vi "syringe_pump_tester.vi"() -> ()   [LabVIEW 2018]
panel:
  in  "Max Pull":bool
  in  "Max Push":bool
  in  "Stop Hold":bool
  out "System Status":T1={"pumpState"=2, "pumpError"=0, "suppliedVolume_ml"=nan, "flowRate_mlmin"=0.0}
  in  "Flow Config":T2={"direction"=1, "desVolume_ml"=5.0, "desFlowrate_mlpmin"=5.0, "syringeDiameter_mm"=20.0}
  in  "Hardware Config":T3={"pwmFrequency"=0, "pwmSlope"=0, "pwmJitter"=0, "stepMode"=32, "maxDriverCurrent_mA"=850, "stepsPerRev"=400, "leadScrewPitch_mm"=1.5, "maxPullPushAcc_RevPerSecSec"=4.0, "maxPullPushVel_RevPerSec"=4.0, "pumpAcc_RevPerSecSec"=0.1, "pumpDec_RevPerSecSec"=0.1}
  in  "Apply Hardware Config":bool
  in  "Apply Flow Config":bool
  in  "Stop Pump":bool
  in  "Start Pump":bool
  out "Error Code":T4(ring)
  out "Return FID":u8=1
  out "FID":u8=1
  in  "IP Address":string="192.168.5.104"
  out "error out":errorcluster={"status"=TRUE, "code"=56, "source"="TCP Open Connection in syringe_pump_tester.vi"}
  in  "Get System Status":bool
  in  "Stop":bool
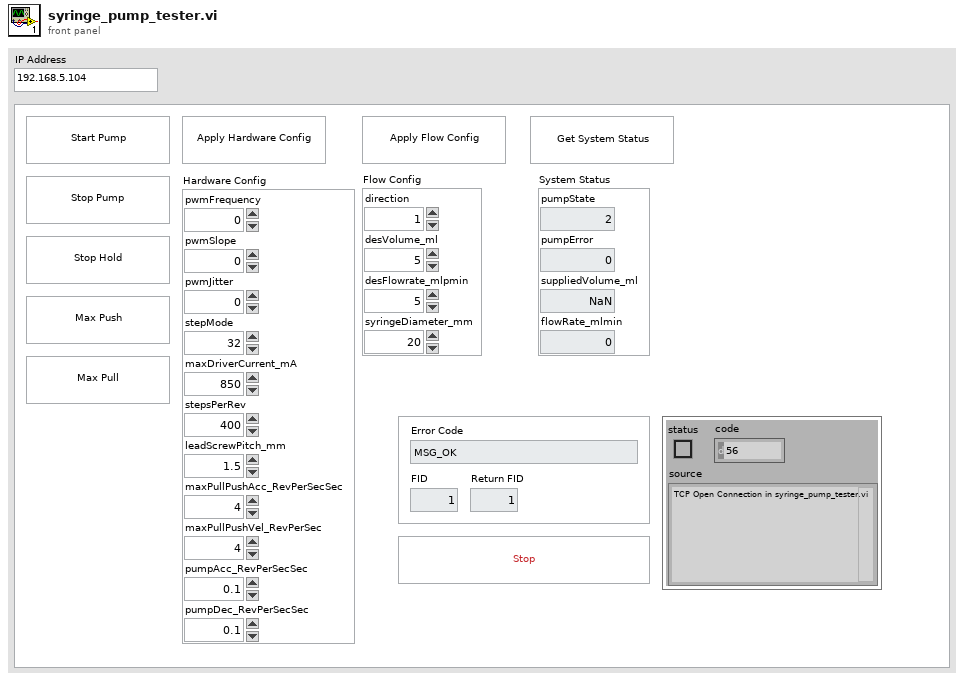
[diagram p1: front panel]
types:
  T1 = cluster{"pumpState":i32, "pumpError":i32, "suppliedVolume_ml":sgl, "flowRate_mlmin":sgl}
  T2 = cluster{"direction":u8, "desVolume_ml":sgl, "desFlowrate_mlpmin":sgl, "syringeDiameter_mm":sgl}
  T3 = cluster{"pwmFrequency":u8, "pwmSlope":u8, "pwmJitter":u8, "stepMode":u8, "maxDriverCurrent_mA":u16, "stepsPerRev":i32, "leadScrewPitch_mm":sgl, "maxPullPushAcc_RevPerSecSec":sgl, "maxPullPushVel_RevPerSec":sgl, "pumpAcc_RevPerSecSec":sgl, "pumpDec_RevPerSecSec":sgl}
  T4 = enum16{"MSG_OK", "MSG_ERROR_INVALID_PARAMETER", "MSG_ERROR_NOT_SUPPORTED", "MSG_ERROR_PUMP_RUNNING", "MSG_ERROR_CHECK_POWER", "MSG_ERROR_FLOW_NOT_CONFIGURED", "MSG_ERROR_STEPDRV_NOT_CONFIGURED", "MSG_ERROR_LIMIT_SW_ACTIVE", "MSG_ERROR_STEPDRV_ERROR", "MSG_ERROR_NO_I2C_COM", "MSG_ERROR_SWITCHING_OVER_MAX"}
  T5 = enum16{"big-endian, network order", "native, host order", "little-endian"}
  T6 = cluster{"connection ID":refnum<k5>, "header length":i32}
  T7 = cluster{"header":cluster{"length":u8, "fid":u8, "error":u8}}
  T8 = cluster{"header":cluster{"length":u8, "fid":u8, "error":u8}, "Hardware Config":cluster{"pwmFrequency":u8, "pwmSlope":u8, "pwmJitter":u8, "stepMode":u8, "maxDriverCurrent_mA":u16, "stepsPerRev":i32, "leadScrewPitch_mm":sgl, "maxPullPushAcc_RevPerSecSec":sgl, "maxPullPushVel_RevPerSec":sgl, "pumpAcc_RevPerSecSec":sgl, "pumpDec_RevPerSecSec":sgl}}
  T9 = cluster{"header":cluster{"length":u8, "fid":u8, "error":u8}, "Flow Config":cluster{"direction":u8, "desVolume_ml":sgl, "desFlowrate_mlpmin":sgl, "syringeDiameter_mm":sgl}}
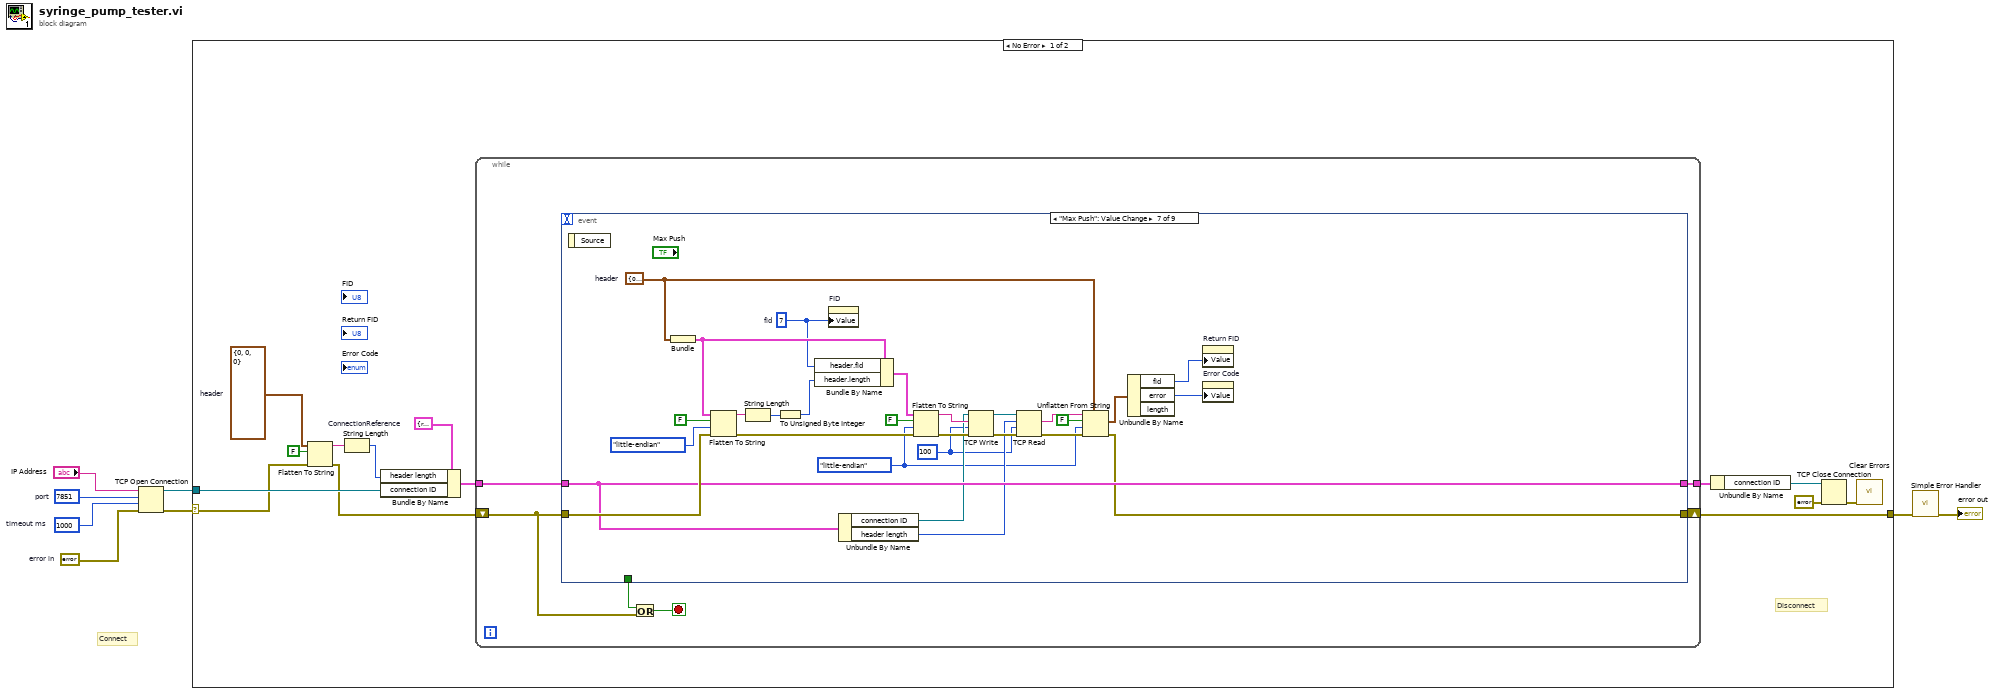
[diagram p0: block diagram]
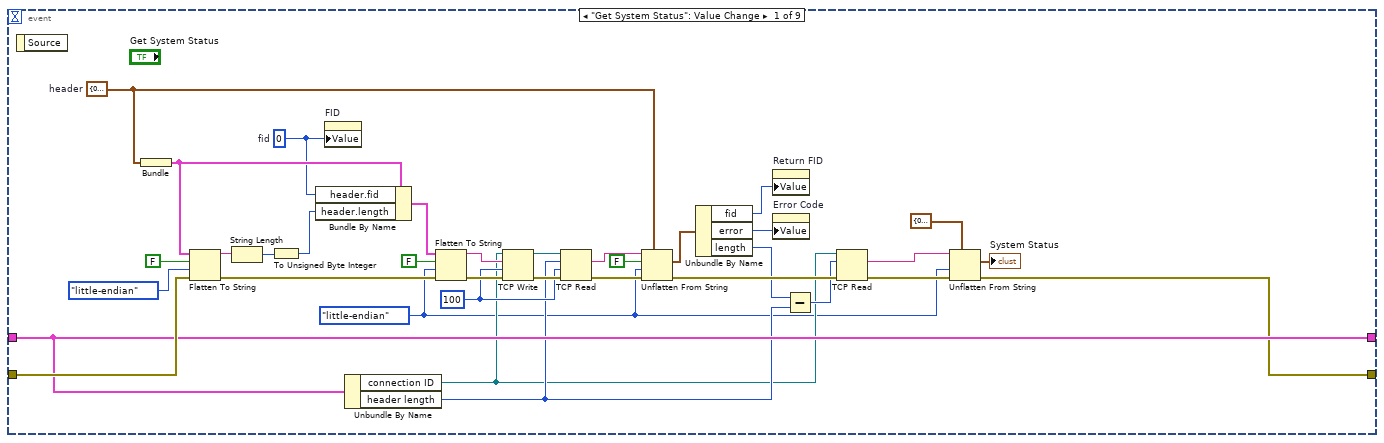
[diagram p2: hidden frame]
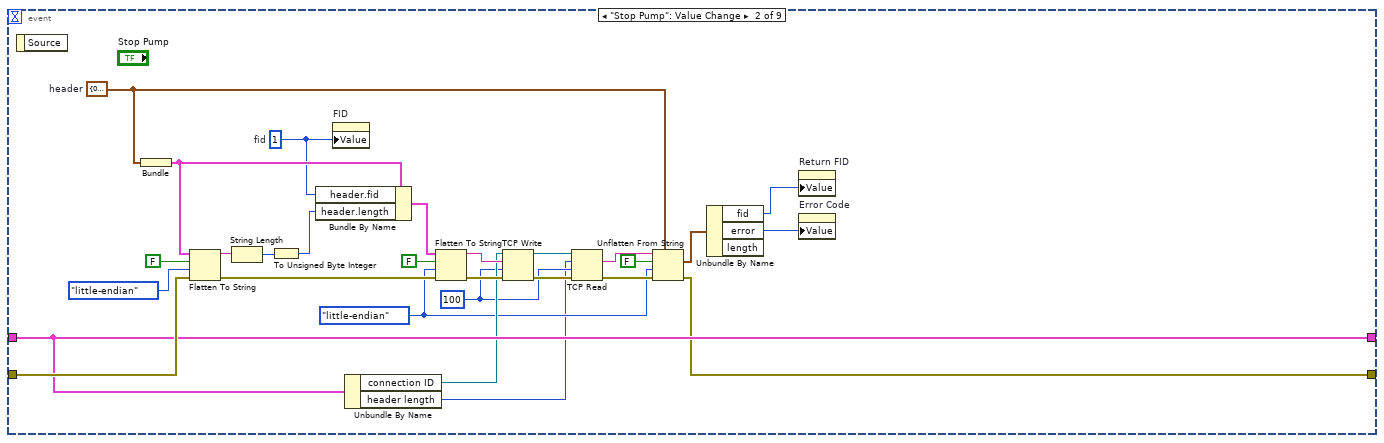
[diagram p3: hidden frame]
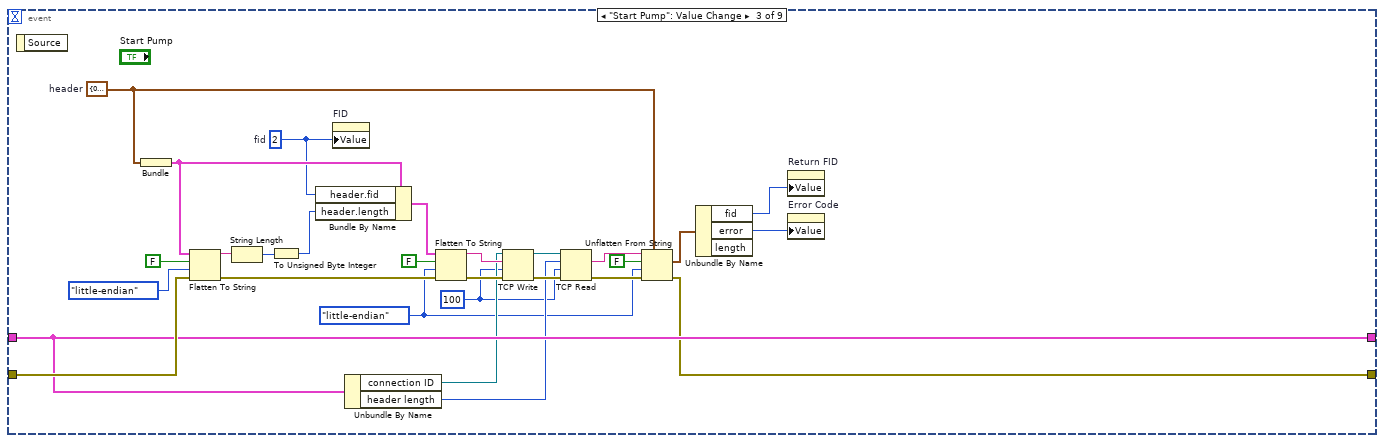
[diagram p4: hidden frame]
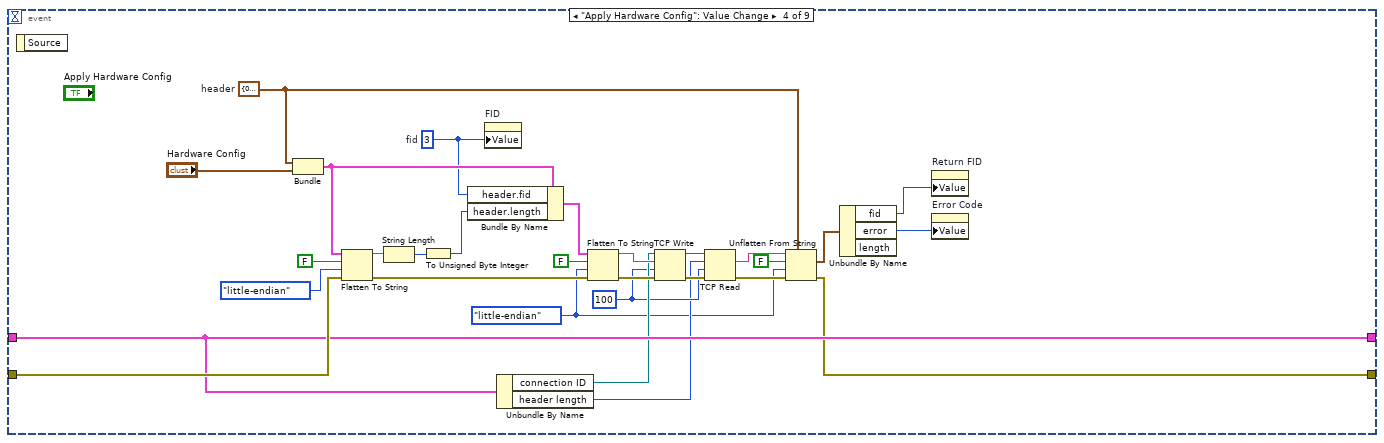
[diagram p5: hidden frame]
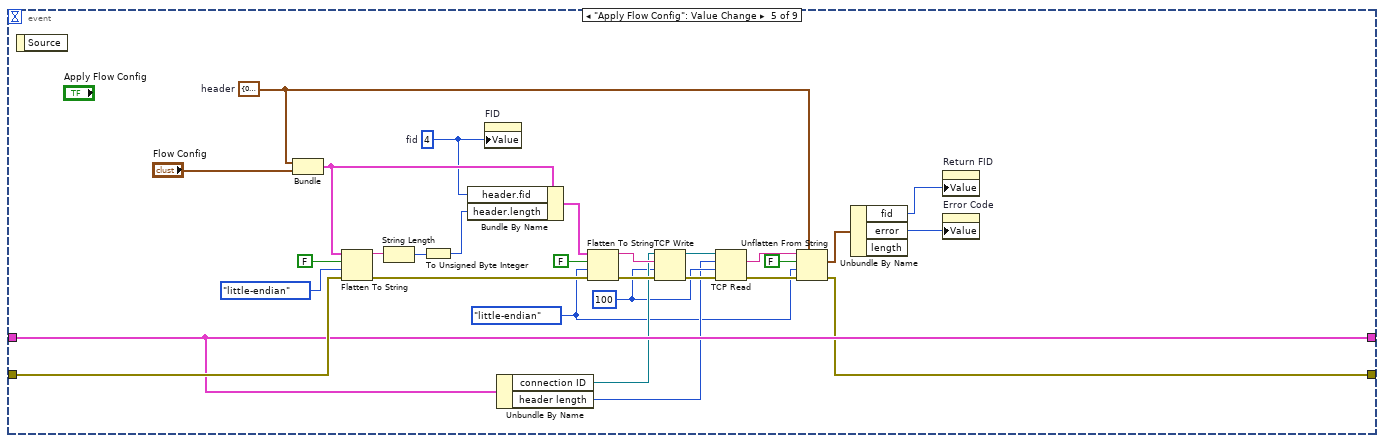
[diagram p6: hidden frame]
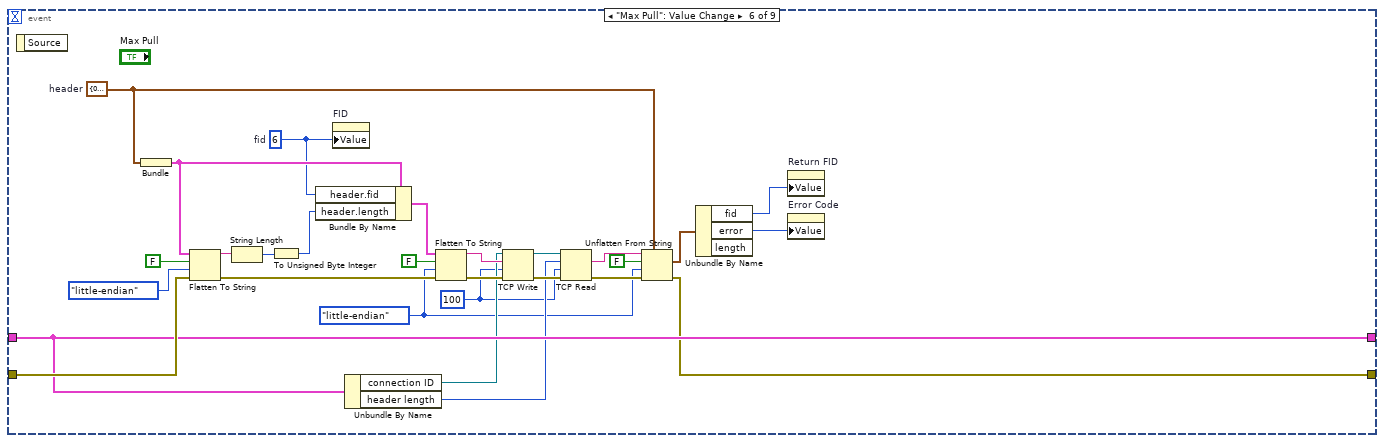
[diagram p7: hidden frame]
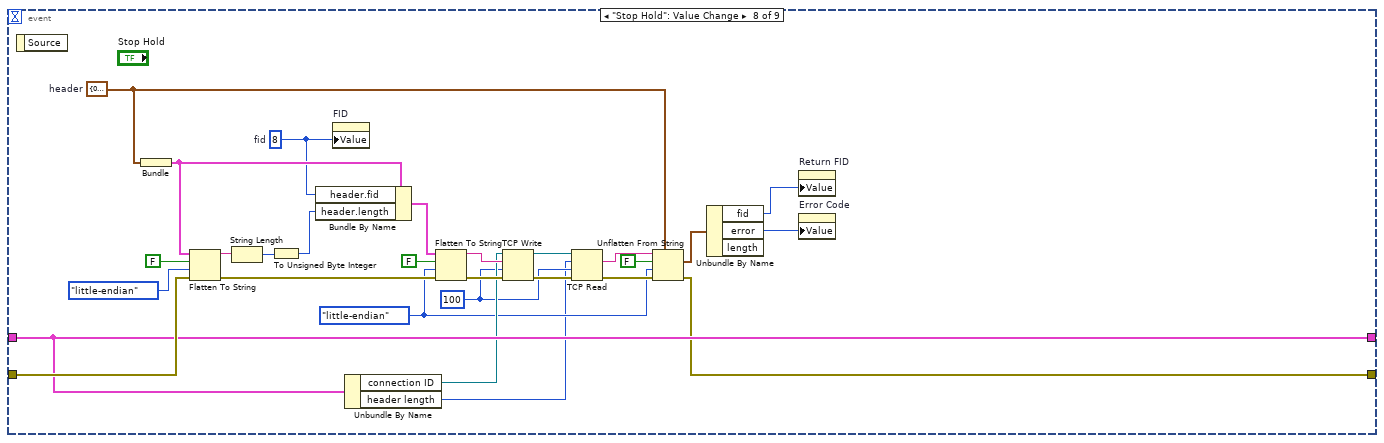
[diagram p8: hidden frame]
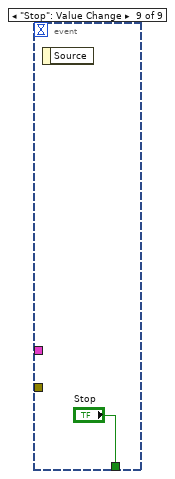
[diagram p9: hidden frame]
diagram:
  w6 = errorcluster {"status"=FALSE, "code"=0, "source"=""}  # error in
  w7 = 1000  # timeout ms
  w8 = u16 7851  # port
  # "Connect"
  n1 = TCP Open Connection(address="IP Address", remote port or service name=w8, timeout ms (60000)=w7, error in (no error)=w6) -> (connection ID=w5:refnum<k5>, error out=w1:errorcluster)  [unwired: 1 in]
  n2 = case shown="No Error" w1 {
    selector: w1 -> [w9 w263]
    tunnel: w5 -> [w18 _]
    tunnel: [w10 w263] -> w2
    frame No Error {
      w17 = cluster{"length":u8, "fid":u8, "error":u8} {"length"=0, "fid"=0, "error"=0}  # header
      w19 = T6 {"connection ID"=refnum, "header length"=0}  # ConnectionReference
      # "Disconnect"
      n3 = Flatten To String(anything=w17, prepend array or string size? (T)=FALSE, error in (no error)=w9) -> (data string=w15:string, error out=w11:errorcluster)  [unwired: 1 in, 1 out]
      n4 = String Length(string=w15) -> (length=w14:i32)
      n5 = Bundle By Name(cluster=w19, "header length"=w14, "connection ID"=w18) -> (w13:T6)
      n6 = while {
        tunnel: w13 -> [w28]
        tunnel: [w27] -> w12
        shift-right: [w26] -> w10
        shift-left: w11 -> [w24]
        stop <- w25 stop-if-true
        n7 = event shown="[6] \"Max Push\": Value Change" {
          selector: _ -> [_ _ _ _ _ _ _ _ _]
          dyn-events: _ -> [_ _ _ _ _ _ _ _ _]
          timeout: _ -> [_ _ _ _ _ _ _ _ _]
          tunnel: w28 -> [w52 w80 w108 w137 w166 w194 w222 w250 _]
          tunnel: [w52 w80 w108 w137 w166 w194 w222 w250 _] -> w27
          tunnel: w24 -> [w53 w81 w109 w138 w167 w195 w223 w251 _]
          tunnel: [w35 w71 w92 w123 w150 w178 w206 w241 _] -> w26
          tunnel: [_ _ _ _ _ _ _ _ "Stop"] -> w23
          event "Get System Status": Value Change {
            w44 = cluster{"length":u8, "fid":u8, "error":u8} {"length"=0, "fid"=0, "error"=0}  # header
            w46 = 100 ("timeout ms (25000)")
            w32 = u8 0  # fid
            w34 = T5."little-endian" ("byte order (0:big-endian, network order)")
            n8 = event-data() -> ()  [unwired: 1 in, 1 out]
            n9 = Bundle("header"=w44) -> (w59:T7)  [unwired: 1 in]
            n10 = Flatten To String(anything=w59, prepend array or string size? (T)=FALSE, byte order (0:big-endian, network order)=T5."little-endian", error in (no error)=w53) -> (data string=w57:string, error out=w58:errorcluster)  [unwired: 1 out]
            n11 = String Length(string=w57) -> (length=w56:i32)
            n12 = To Unsigned Byte Integer(number=w56) -> (unsigned 8bit integer=w55:u8)
            n13 = Bundle By Name(cluster=w59, "header.fid"=w32, "header.length"=w55) -> (w60:T7)
            n14 = property on="FID" class="DigNum (strict)"("Value"=w32) -> ()  [unwired: 2 in, 2 out]
            n15 = Unbundle By Name(w52) -> ("connection ID"=w38:refnum<k5>, "header length"=w40:i32)
            n16 = Flatten To String(anything=w60, prepend array or string size? (T)=FALSE, byte order (0:big-endian, network order)=w34, error in (no error)=w58) -> (data string=w62:string, error out=w63:errorcluster)  [unwired: 1 out]
            n17 = TCP Write(connection ID=w38, data in=w62, error in (no error)=w63, 9:w46) -> (connection ID out=w47:refnum<k5>, error out=w48:errorcluster)  [unwired: 1 out]
            n18 = TCP Read(connection ID=w47, bytes to read=w40, error in (no error)=w48, 9:w46) -> (data out=w49:string, error out=w50:errorcluster)  [unwired: 1 in, 1 out]
            n19 = Unflatten From String(type=w44, binary string=w49, data includes array or string size? (T)=FALSE, byte order (0:big-endian, network order)=w34, error in (no error)=w50) -> (value=w45:cluster{"length":u8, "fid":u8, "error":u8}, error out=w42:errorcluster)  [unwired: 1 out]
            n20 = Unbundle By Name(w45) -> ("fid"=w33:u8, "error"=w31:u8, "length"=w41:u8)
            n21 = property on="Return FID" class="DigNum (strict)"("Value"=w33) -> ()  [unwired: 2 in, 2 out]
            n22 = property on="Error Code" class="Enum (strict)"("Value"=w31) -> ()  [unwired: 2 in, 2 out]
            n23 = Subtract(x=w41, y=w40) -> (x-y=w39:i32)
            n24 = TCP Read(connection ID=w38, bytes to read=w39, error in (no error)=w42) -> (data out=w37:string, error out=w36:errorcluster)  [unwired: 2 in, 1 out]
            n25 = Unflatten From String(type=T1 {"pumpState"=0, "pumpError"=0, "suppliedVolume_ml"=0.0, "flowRate_mlmin"=0.0} ("system status"), binary string=w37, byte order (0:big-endian, network order)=w34, error in (no error)=w36) -> (value=→"System Status":T1, error out=w35:errorcluster)  [unwired: 1 in, 1 out]
          }
          event "Stop Pump": Value Change {
            w70 = cluster{"length":u8, "fid":u8, "error":u8} {"length"=0, "fid"=0, "error"=0}  # header
            w68 = 100 ("timeout ms (25000)")
            w77 = u8 1  # fid
            w69 = T5."little-endian" ("byte order (0:big-endian, network order)")
            n26 = event-data() -> ()  [unwired: 1 in, 1 out]
            n27 = Bundle("header"=w70) -> (w87:T7)  [unwired: 1 in]
            n28 = Flatten To String(anything=w87, prepend array or string size? (T)=FALSE, byte order (0:big-endian, network order)=T5."little-endian", error in (no error)=w81) -> (data string=w85:string, error out=w86:errorcluster)  [unwired: 1 out]
            n29 = String Length(string=w85) -> (length=w84:i32)
            n30 = To Unsigned Byte Integer(number=w84) -> (unsigned 8bit integer=w83:u8)
            n31 = Bundle By Name(cluster=w87, "header.fid"=w77, "header.length"=w83) -> (w88:T7)
            n32 = property on="FID" class="DigNum (strict)"("Value"=w77) -> ()  [unwired: 2 in, 2 out]
            n33 = Unbundle By Name(w80) -> ("connection ID"=w78:refnum<k5>, "header length"=w67:i32)
            n34 = Flatten To String(anything=w88, prepend array or string size? (T)=FALSE, byte order (0:big-endian, network order)=w69, error in (no error)=w86) -> (data string=w90:string, error out=w91:errorcluster)  [unwired: 1 out]
            n35 = TCP Write(connection ID=w78, data in=w90, error in (no error)=w91, 9:w68) -> (connection ID out=w66:refnum<k5>, error out=w73:errorcluster)  [unwired: 1 out]
            n36 = TCP Read(connection ID=w66, bytes to read=w67, error in (no error)=w73, 9:w68) -> (data out=w76:string, error out=w72:errorcluster)  [unwired: 1 in, 1 out]
            n37 = Unflatten From String(type=w70, binary string=w76, data includes array or string size? (T)=FALSE, byte order (0:big-endian, network order)=w69, error in (no error)=w72) -> (value=w75:cluster{"length":u8, "fid":u8, "error":u8}, error out=w71:errorcluster)  [unwired: 1 out]
            n38 = Unbundle By Name(w75) -> ("fid"=w65:u8, "error"=w64:u8)  [unwired: 1 out]
            n39 = property on="Return FID" class="DigNum (strict)"("Value"=w65) -> ()  [unwired: 2 in, 2 out]
            n40 = property on="Error Code" class="Enum (strict)"("Value"=w64) -> ()  [unwired: 2 in, 2 out]
          }
          event "Start Pump": Value Change {
            w101 = cluster{"length":u8, "fid":u8, "error":u8} {"length"=0, "fid"=0, "error"=0}  # header
            w93 = 100 ("timeout ms (25000)")
            w97 = u8 2  # fid
            w94 = T5."little-endian" ("byte order (0:big-endian, network order)")
            n41 = event-data() -> ()  [unwired: 1 in, 1 out]
            n42 = Bundle("header"=w101) -> (w115:T7)  [unwired: 1 in]
            n43 = Flatten To String(anything=w115, prepend array or string size? (T)=FALSE, byte order (0:big-endian, network order)=T5."little-endian", error in (no error)=w109) -> (data string=w113:string, error out=w114:errorcluster)  [unwired: 1 out]
            n44 = String Length(string=w113) -> (length=w112:i32)
            n45 = To Unsigned Byte Integer(number=w112) -> (unsigned 8bit integer=w111:u8)
            n46 = Bundle By Name(cluster=w115, "header.fid"=w97, "header.length"=w111) -> (w116:T7)
            n47 = property on="FID" class="DigNum (strict)"("Value"=w97) -> ()  [unwired: 2 in, 2 out]
            n48 = Unbundle By Name(w108) -> ("connection ID"=w98:refnum<k5>, "header length"=w99:i32)
            n49 = Flatten To String(anything=w116, prepend array or string size? (T)=FALSE, byte order (0:big-endian, network order)=w94, error in (no error)=w114) -> (data string=w118:string, error out=w119:errorcluster)  [unwired: 1 out]
            n50 = TCP Write(connection ID=w98, data in=w118, error in (no error)=w119, 9:w93) -> (connection ID out=w103:refnum<k5>, error out=w104:errorcluster)  [unwired: 1 out]
            n51 = TCP Read(connection ID=w103, bytes to read=w99, error in (no error)=w104, 9:w93) -> (data out=w105:string, error out=w106:errorcluster)  [unwired: 1 in, 1 out]
            n52 = Unflatten From String(type=w101, binary string=w105, data includes array or string size? (T)=FALSE, byte order (0:big-endian, network order)=w94, error in (no error)=w106) -> (value=w102:cluster{"length":u8, "fid":u8, "error":u8}, error out=w92:errorcluster)  [unwired: 1 out]
            n53 = Unbundle By Name(w102) -> ("fid"=w96:u8, "error"=w95:u8)  [unwired: 1 out]
            n54 = property on="Return FID" class="DigNum (strict)"("Value"=w96) -> ()  [unwired: 2 in, 2 out]
            n55 = property on="Error Code" class="Enum (strict)"("Value"=w95) -> ()  [unwired: 2 in, 2 out]
          }
          event "Apply Hardware Config": Value Change {
            w126 = cluster{"length":u8, "fid":u8, "error":u8} {"length"=0, "fid"=0, "error"=0}  # header
            w127 = 100 ("timeout ms (25000)")
            w134 = u8 3  # fid
            w120 = T5."little-endian" ("byte order (0:big-endian, network order)")
            n56 = event-data() -> ()  [unwired: 1 in, 1 out]
            n57 = Bundle("header"=w126, "Hardware Config"="Hardware Config") -> (w144:T8)  [unwired: 1 in]
            n58 = Flatten To String(anything=w144, prepend array or string size? (T)=FALSE, byte order (0:big-endian, network order)=T5."little-endian", error in (no error)=w138) -> (data string=w142:string, error out=w143:errorcluster)  [unwired: 1 out]
            n59 = String Length(string=w142) -> (length=w141:i32)
            n60 = To Unsigned Byte Integer(number=w141) -> (unsigned 8bit integer=w140:u8)
            n61 = Bundle By Name(cluster=w144, "header.fid"=w134, "header.length"=w140) -> (w145:T8)
            n62 = property on="FID" class="DigNum (strict)"("Value"=w134) -> ()  [unwired: 2 in, 2 out]
            n63 = Unbundle By Name(w137) -> ("connection ID"=w135:refnum<k5>, "header length"=w124:i32)
            n64 = Flatten To String(anything=w145, prepend array or string size? (T)=FALSE, byte order (0:big-endian, network order)=w120, error in (no error)=w143) -> (data string=w147:string, error out=w148:errorcluster)  [unwired: 1 out]
            n65 = TCP Write(connection ID=w135, data in=w147, error in (no error)=w148, 9:w127) -> (connection ID out=w125:refnum<k5>, error out=w128:errorcluster)  [unwired: 1 out]
            n66 = TCP Read(connection ID=w125, bytes to read=w124, error in (no error)=w128, 9:w127) -> (data out=w131:string, error out=w132:errorcluster)  [unwired: 1 in, 1 out]
            n67 = Unflatten From String(type=w126, binary string=w131, data includes array or string size? (T)=FALSE, byte order (0:big-endian, network order)=w120, error in (no error)=w132) -> (value=w130:cluster{"length":u8, "fid":u8, "error":u8}, error out=w123:errorcluster)  [unwired: 1 out]
            n68 = Unbundle By Name(w130) -> ("fid"=w122:u8, "error"=w121:u8)  [unwired: 1 out]
            n69 = property on="Return FID" class="DigNum (strict)"("Value"=w122) -> ()  [unwired: 2 in, 2 out]
            n70 = property on="Error Code" class="Enum (strict)"("Value"=w121) -> ()  [unwired: 2 in, 2 out]
          }
          event "Apply Flow Config": Value Change {
            w153 = cluster{"length":u8, "fid":u8, "error":u8} {"length"=0, "fid"=0, "error"=0}  # header
            w156 = 100 ("timeout ms (25000)")
            w163 = u8 4  # fid
            w149 = T5."little-endian" ("byte order (0:big-endian, network order)")
            n71 = event-data() -> ()  [unwired: 1 in, 1 out]
            n72 = Bundle("header"=w153, "Flow Config"="Flow Config") -> (w173:T9)  [unwired: 1 in]
            n73 = Flatten To String(anything=w173, prepend array or string size? (T)=FALSE, byte order (0:big-endian, network order)=T5."little-endian", error in (no error)=w167) -> (data string=w171:string, error out=w172:errorcluster)  [unwired: 1 out]
            n74 = String Length(string=w171) -> (length=w170:i32)
            n75 = To Unsigned Byte Integer(number=w170) -> (unsigned 8bit integer=w169:u8)
            n76 = Bundle By Name(cluster=w173, "header.fid"=w163, "header.length"=w169) -> (w174:T9)
            n77 = property on="FID" class="DigNum (strict)"("Value"=w163) -> ()  [unwired: 2 in, 2 out]
            n78 = Unbundle By Name(w166) -> ("connection ID"=w164:refnum<k5>, "header length"=w155:i32)
            n79 = Flatten To String(anything=w174, prepend array or string size? (T)=FALSE, byte order (0:big-endian, network order)=w149, error in (no error)=w172) -> (data string=w176:string, error out=w177:errorcluster)  [unwired: 1 out]
            n80 = TCP Write(connection ID=w164, data in=w176, error in (no error)=w177, 9:w156) -> (connection ID out=w154:refnum<k5>, error out=w157:errorcluster)  [unwired: 1 out]
            n81 = TCP Read(connection ID=w154, bytes to read=w155, error in (no error)=w157, 9:w156) -> (data out=w160:string, error out=w161:errorcluster)  [unwired: 1 in, 1 out]
            n82 = Unflatten From String(type=w153, binary string=w160, data includes array or string size? (T)=FALSE, byte order (0:big-endian, network order)=w149, error in (no error)=w161) -> (value=w159:cluster{"length":u8, "fid":u8, "error":u8}, error out=w150:errorcluster)  [unwired: 1 out]
            n83 = Unbundle By Name(w159) -> ("fid"=w152:u8, "error"=w151:u8)  [unwired: 1 out]
            n84 = property on="Return FID" class="DigNum (strict)"("Value"=w152) -> ()  [unwired: 2 in, 2 out]
            n85 = property on="Error Code" class="Enum (strict)"("Value"=w151) -> ()  [unwired: 2 in, 2 out]
          }
          event "Max Pull": Value Change {
            w187 = cluster{"length":u8, "fid":u8, "error":u8} {"length"=0, "fid"=0, "error"=0}  # header
            w179 = 100 ("timeout ms (25000)")
            w183 = u8 6  # fid
            w180 = T5."little-endian" ("byte order (0:big-endian, network order)")
            n86 = event-data() -> ()  [unwired: 1 in, 1 out]
            n87 = Bundle("header"=w187) -> (w201:T7)  [unwired: 1 in]
            n88 = Flatten To String(anything=w201, prepend array or string size? (T)=FALSE, byte order (0:big-endian, network order)=T5."little-endian", error in (no error)=w195) -> (data string=w199:string, error out=w200:errorcluster)  [unwired: 1 out]
            n89 = String Length(string=w199) -> (length=w198:i32)
            n90 = To Unsigned Byte Integer(number=w198) -> (unsigned 8bit integer=w197:u8)
            n91 = Bundle By Name(cluster=w201, "header.fid"=w183, "header.length"=w197) -> (w202:T7)
            n92 = property on="FID" class="DigNum (strict)"("Value"=w183) -> ()  [unwired: 2 in, 2 out]
            n93 = Unbundle By Name(w194) -> ("connection ID"=w184:refnum<k5>, "header length"=w185:i32)
            n94 = Flatten To String(anything=w202, prepend array or string size? (T)=FALSE, byte order (0:big-endian, network order)=w180, error in (no error)=w200) -> (data string=w204:string, error out=w205:errorcluster)  [unwired: 1 out]
            n95 = TCP Write(connection ID=w184, data in=w204, error in (no error)=w205, 9:w179) -> (connection ID out=w189:refnum<k5>, error out=w190:errorcluster)  [unwired: 1 out]
            n96 = TCP Read(connection ID=w189, bytes to read=w185, error in (no error)=w190, 9:w179) -> (data out=w191:string, error out=w192:errorcluster)  [unwired: 1 in, 1 out]
            n97 = Unflatten From String(type=w187, binary string=w191, data includes array or string size? (T)=FALSE, byte order (0:big-endian, network order)=w180, error in (no error)=w192) -> (value=w188:cluster{"length":u8, "fid":u8, "error":u8}, error out=w178:errorcluster)  [unwired: 1 out]
            n98 = Unbundle By Name(w188) -> ("fid"=w182:u8, "error"=w181:u8)  [unwired: 1 out]
            n99 = property on="Return FID" class="DigNum (strict)"("Value"=w182) -> ()  [unwired: 2 in, 2 out]
            n100 = property on="Error Code" class="Enum (strict)"("Value"=w181) -> ()  [unwired: 2 in, 2 out]
          }
          event "Max Push": Value Change {
            w215 = cluster{"length":u8, "fid":u8, "error":u8} {"length"=0, "fid"=0, "error"=0}  # header
            w207 = 100 ("timeout ms (25000)")
            w211 = u8 7  # fid
            w208 = T5."little-endian" ("byte order (0:big-endian, network order)")
            n101 = event-data() -> ()  [unwired: 1 in, 1 out]
            n102 = Bundle("header"=w215) -> (w229:T7)  [unwired: 1 in]
            n103 = Flatten To String(anything=w229, prepend array or string size? (T)=FALSE, byte order (0:big-endian, network order)=T5."little-endian", error in (no error)=w223) -> (data string=w227:string, error out=w228:errorcluster)  [unwired: 1 out]
            n104 = String Length(string=w227) -> (length=w226:i32)
            n105 = To Unsigned Byte Integer(number=w226) -> (unsigned 8bit integer=w225:u8)
            n106 = Bundle By Name(cluster=w229, "header.fid"=w211, "header.length"=w225) -> (w230:T7)
            n107 = property on="FID" class="DigNum (strict)"("Value"=w211) -> ()  [unwired: 2 in, 2 out]
            n108 = Unbundle By Name(w222) -> ("connection ID"=w212:refnum<k5>, "header length"=w213:i32)
            n109 = Flatten To String(anything=w230, prepend array or string size? (T)=FALSE, byte order (0:big-endian, network order)=w208, error in (no error)=w228) -> (data string=w232:string, error out=w233:errorcluster)  [unwired: 1 out]
            n110 = TCP Write(connection ID=w212, data in=w232, error in (no error)=w233, 9:w207) -> (connection ID out=w217:refnum<k5>, error out=w218:errorcluster)  [unwired: 1 out]
            n111 = TCP Read(connection ID=w217, bytes to read=w213, error in (no error)=w218, 9:w207) -> (data out=w219:string, error out=w220:errorcluster)  [unwired: 1 in, 1 out]
            n112 = Unflatten From String(type=w215, binary string=w219, data includes array or string size? (T)=FALSE, byte order (0:big-endian, network order)=w208, error in (no error)=w220) -> (value=w216:cluster{"length":u8, "fid":u8, "error":u8}, error out=w206:errorcluster)  [unwired: 1 out]
            n113 = Unbundle By Name(w216) -> ("fid"=w210:u8, "error"=w209:u8)  [unwired: 1 out]
            n114 = property on="Return FID" class="DigNum (strict)"("Value"=w210) -> ()  [unwired: 2 in, 2 out]
            n115 = property on="Error Code" class="Enum (strict)"("Value"=w209) -> ()  [unwired: 2 in, 2 out]
          }
          event "Stop Hold": Value Change {
            w240 = cluster{"length":u8, "fid":u8, "error":u8} {"length"=0, "fid"=0, "error"=0}  # header
            w238 = 100 ("timeout ms (25000)")
            w247 = u8 8  # fid
            w239 = T5."little-endian" ("byte order (0:big-endian, network order)")
            n116 = event-data() -> ()  [unwired: 1 in, 1 out]
            n117 = Bundle("header"=w240) -> (w257:T7)  [unwired: 1 in]
            n118 = Flatten To String(anything=w257, prepend array or string size? (T)=FALSE, byte order (0:big-endian, network order)=T5."little-endian", error in (no error)=w251) -> (data string=w255:string, error out=w256:errorcluster)  [unwired: 1 out]
            n119 = String Length(string=w255) -> (length=w254:i32)
            n120 = To Unsigned Byte Integer(number=w254) -> (unsigned 8bit integer=w253:u8)
            n121 = Bundle By Name(cluster=w257, "header.fid"=w247, "header.length"=w253) -> (w258:T7)
            n122 = property on="FID" class="DigNum (strict)"("Value"=w247) -> ()  [unwired: 2 in, 2 out]
            n123 = Unbundle By Name(w250) -> ("connection ID"=w248:refnum<k5>, "header length"=w237:i32)
            n124 = Flatten To String(anything=w258, prepend array or string size? (T)=FALSE, byte order (0:big-endian, network order)=w239, error in (no error)=w256) -> (data string=w260:string, error out=w261:errorcluster)  [unwired: 1 out]
            n125 = TCP Write(connection ID=w248, data in=w260, error in (no error)=w261, 9:w238) -> (connection ID out=w236:refnum<k5>, error out=w243:errorcluster)  [unwired: 1 out]
            n126 = TCP Read(connection ID=w236, bytes to read=w237, error in (no error)=w243, 9:w238) -> (data out=w246:string, error out=w242:errorcluster)  [unwired: 1 in, 1 out]
            n127 = Unflatten From String(type=w240, binary string=w246, data includes array or string size? (T)=FALSE, byte order (0:big-endian, network order)=w239, error in (no error)=w242) -> (value=w245:cluster{"length":u8, "fid":u8, "error":u8}, error out=w241:errorcluster)  [unwired: 1 out]
            n128 = Unbundle By Name(w245) -> ("fid"=w235:u8, "error"=w234:u8)  [unwired: 1 out]
            n129 = property on="Return FID" class="DigNum (strict)"("Value"=w235) -> ()  [unwired: 2 in, 2 out]
            n130 = property on="Error Code" class="Enum (strict)"("Value"=w234) -> ()  [unwired: 2 in, 2 out]
          }
          event "Stop": Value Change {
            n131 = event-data() -> ()  [unwired: 1 in, 1 out]
          }
        }
        n132 = Or(x=w23, y=w24) -> (x .or. y?=w25:bool)
      }
      n133 = Unbundle By Name(w12) -> ("connection ID"=w20:refnum<k5>)
      n134 = TCP Close Connection(connection ID=w20, error in (no error)=errorcluster {"status"=FALSE, "code"=0, "source"=""}) -> (error out=w21:errorcluster)  [unwired: 1 in, 1 out]
      n135 = call <vilib>:"Clear Errors.vi"("error in (no error)"=w21) -> ()  [unwired: 5 in, 2 out]
    }
    frame Error {
    }
  }
  n136 = call <vilib>:"Simple Error Handler.vi"("error in (no error)"=w2) -> ("error out"=→"error out":errorcluster)  [unwired: 4 in, 4 out]
